vi "New.vi"(8 "error in (no error)":errorcluster, 10 "Error data (JSON)":T1={"Request ID"=0, "Message type that caused error"=enum."HELLO", "Error/Abort details (JSON)"={"URI"="", "Arguments Payload"="", "ArgumentKw Payload"="{}", "Details"="{}", "Associated LabVIEW Error"={"status"=FALSE, "code"=0, "source"=""}}}) -> (0 "error out":errorcluster, 3 "Error JSON2 out":refnum<class "Error JSON.lvclass">)   [LabVIEW 2020, in "wamplv.lvlib" / "Error JSON.lvclass"]
uses:
  Error JSON.lvclass
  WAMP Client/API/TypeDefs/Error or abort detail (JSON).ctl
  wamplv.lvlib
  TypeDefs/WAMP Message Codes.ctl
  WAMP Client/Private/TypeDef/Error (JSON).ctl
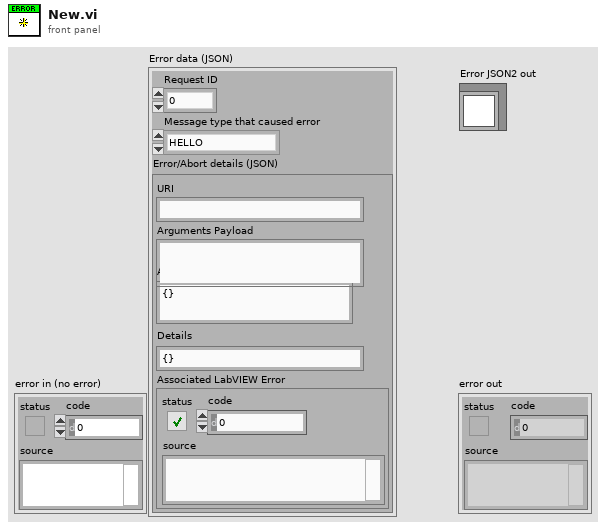
[diagram p1: front panel]
types:
  T1 = typedef "wamplv.lvlib/Error (JSON).ctl" = cluster{"Request ID":u64, "Message type that caused error":T2, "Error/Abort details (JSON)":T3}
  T2 = typedef "wamplv.lvlib/WAMP Message Codes.ctl" = enum8{"HELLO", "WELCOME", "CHALLENGE", "AUTHENTICATE", "ABORT", "GOODBYE", "ERROR", "PUBLISH", "PUBLISHED", "SUBSCRIBE", "SUBSCRIBED", "UNSUBSCRIBE", "UNSUBSCRIBED", "EVENT", "CALL", "RESULT", "REGISTER", "REGISTERED", "UNREGISTER", "UNREGISTERED", "INVOCATION", "YIELD"}
  T3 = typedef "wamplv.lvlib/Error or abort detail (JSON).ctl" = cluster{"URI":string, "Arguments Payload":string, "ArgumentKw Payload":string, "Details":string, "Associated LabVIEW Error":errorcluster}
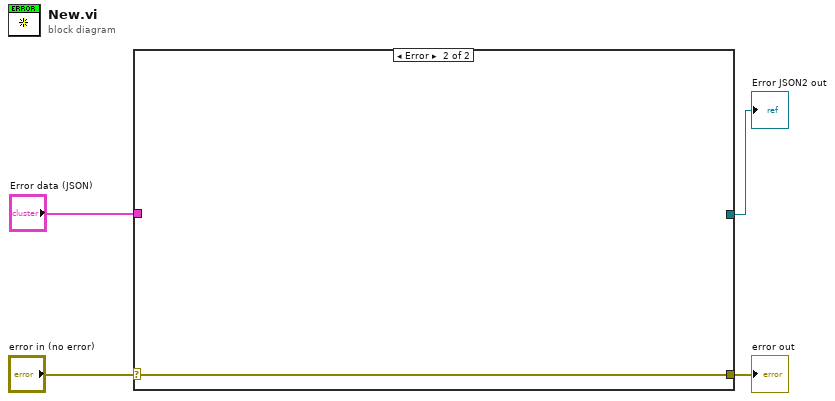
[diagram p0: block diagram]
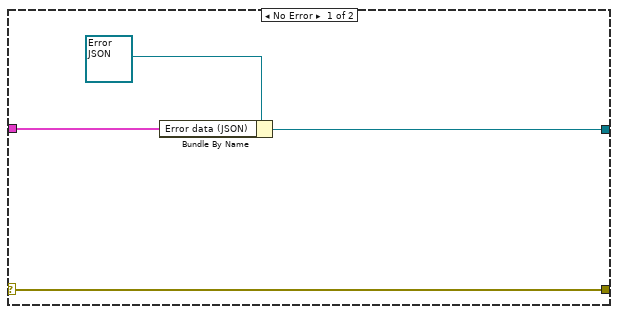
[diagram p2: hidden frame]
diagram:
  n1 = case shown="Error" "error in (no error)" {
    selector: "error in (no error)" -> [w8 w9]
    tunnel: [w8 w9] -> w3
    tunnel: "Error data (JSON)" -> [w7 _]
    tunnel: [w5 _] -> w1
    frame No Error {
      n2 = Bundle By Name(cluster=refnum<class "Error JSON.lvclass"> refnum ("wamplv.lvlib:Error JSON2.lvclass"), "Error data (JSON)"=w7) -> (w5:refnum<class "Error JSON.lvclass">)
    }
    frame Error {
    }
  }
  "error out" <- w3
  "Error JSON2 out" <- w1
